vi "Main.vi"() -> ()   [LabVIEW 2017]
panel:
  out "spreadsheet string":string
  in  "Question 32":enum32{"1", "2", "3", "4", " IDK"}(radio)=enum." IDK"
  in  "Question 31":enum32{"1", "2", "3", "4", " IDK"}(radio)=enum." IDK"
  in  "Question 30":enum32{"1", "2", "3", "4", " IDK"}(radio)=enum." IDK"
  in  "Question 29":enum32{"1", "2", "3", "4", " IDK"}(radio)=enum." IDK"
  in  "Question 28":enum32{"1", "2", "3", "4", " IDK"}(radio)=enum." IDK"
  in  "Question 27":enum32{"1", "2", "3", "4", " IDK"}(radio)=enum." IDK"
  in  "Question 26":enum32{"1", "2", "3", "4", " IDK"}(radio)=enum." IDK"
  in  "Question 25":enum32{"1", "2", "3", "4", " IDK"}(radio)=enum." IDK"
  in  "Question 24":enum32{"1", "2", "3", "4", " IDK"}(radio)=enum." IDK"
  in  "Question 23":enum32{"1", "2", "3", "4", " IDK"}(radio)=enum." IDK"
  in  "Question 22":enum32{"1", "2", "3", "4", " IDK"}(radio)=enum." IDK"
  in  "Question 21":enum32{"1", "2", "3", "4", " IDK"}(radio)=enum." IDK"
  in  "Question 20":enum32{"1", "2", "3", "4", " IDK"}(radio)=enum." IDK"
  in  "Question 19":enum32{"1", "2", "3", "4", " IDK"}(radio)=enum." IDK"
  in  "Question 18":enum32{"1", "2", "3", "4", " IDK"}(radio)=enum." IDK"
  in  "Question 17":enum32{"1", "2", "3", "4", " IDK"}(radio)=enum." IDK"
  in  "Question 16":enum32{"1", "2", "3", "4", " IDK"}(radio)=enum." IDK"
  in  "Question 15":enum32{"1", "2", "3", "4", " IDK"}(radio)=enum." IDK"
  in  "Question 14":enum32{"1", "2", "3", "4", " IDK"}(radio)=enum." IDK"
  in  "Question 13":enum32{"1", "2", "3", "4", " IDK"}(radio)=enum." IDK"
  in  "Question 12":enum32{"1", "2", "3", "4", " IDK"}(radio)=enum." IDK"
  in  "Question 11":enum32{"1", "2", "3", "4", " IDK"}(radio)=enum." IDK"
  in  "Question 10":enum32{"1", "2", "3", "4", " IDK"}(radio)=enum." IDK"
  in  "Question 9":enum32{"1", "2", "3", "4", " IDK"}(radio)=enum." IDK"
  in  "Question 8":enum32{"1", "2", "3", "4", " IDK"}(radio)=enum." IDK"
  in  "Question 7":enum32{"1", "2", "3", "4", " IDK"}(radio)=enum." IDK"
  in  "Question 6":enum32{"1", "2", "3", "4", " IDK"}(radio)=enum." IDK"
  in  "Question 5":enum32{"1", "2", "3", "4", " IDK"}(radio)=enum." IDK"
  in  "Question 4":enum32{"1", "2", "3", "4", " IDK"}(radio)=enum." IDK"
  in  "Question 3":enum32{"1", "2", "3", "4", " IDK"}(radio)=enum." IDK"
  in  "Question 2":enum32{"1", "2", "3", "4", " IDK"}(radio)=enum." IDK"
  in  "VISA resource name":refnum<visa-resource-name>
  in  "Question 1":enum32{"1", "2", "3", "4", " IDK"}(radio)=enum." IDK"
  in  "OK":bool
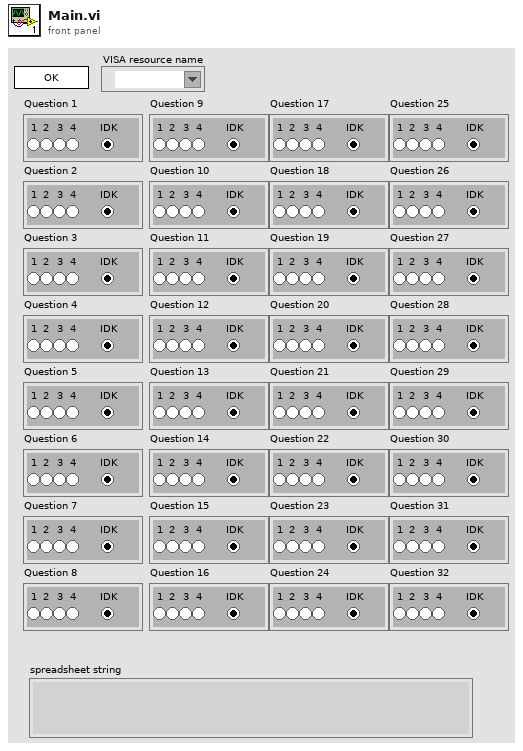
[diagram p1: front panel]
types:
  T1 = enum32{"invalid app kind", "Development System", "Run Time System", "Student Edition", "Embedded LabVIEW", "Evaluation", "Custom"}
  T2 = enum32{"Invalid", "Standard", "Closed", "Hidden", "Minimized", "Maximized"}
  T3 = cluster{"Core":cluster{"Current VI Reference":refnum<vi>, "Close Panel on Exit?":bool}, "Your Boolean data":bool, "Your string data":string, "resource name":refnum<visa-resource-name>}
  T4 = cluster{"Current VI Reference":refnum<vi>, "Close Panel on Exit?":bool}
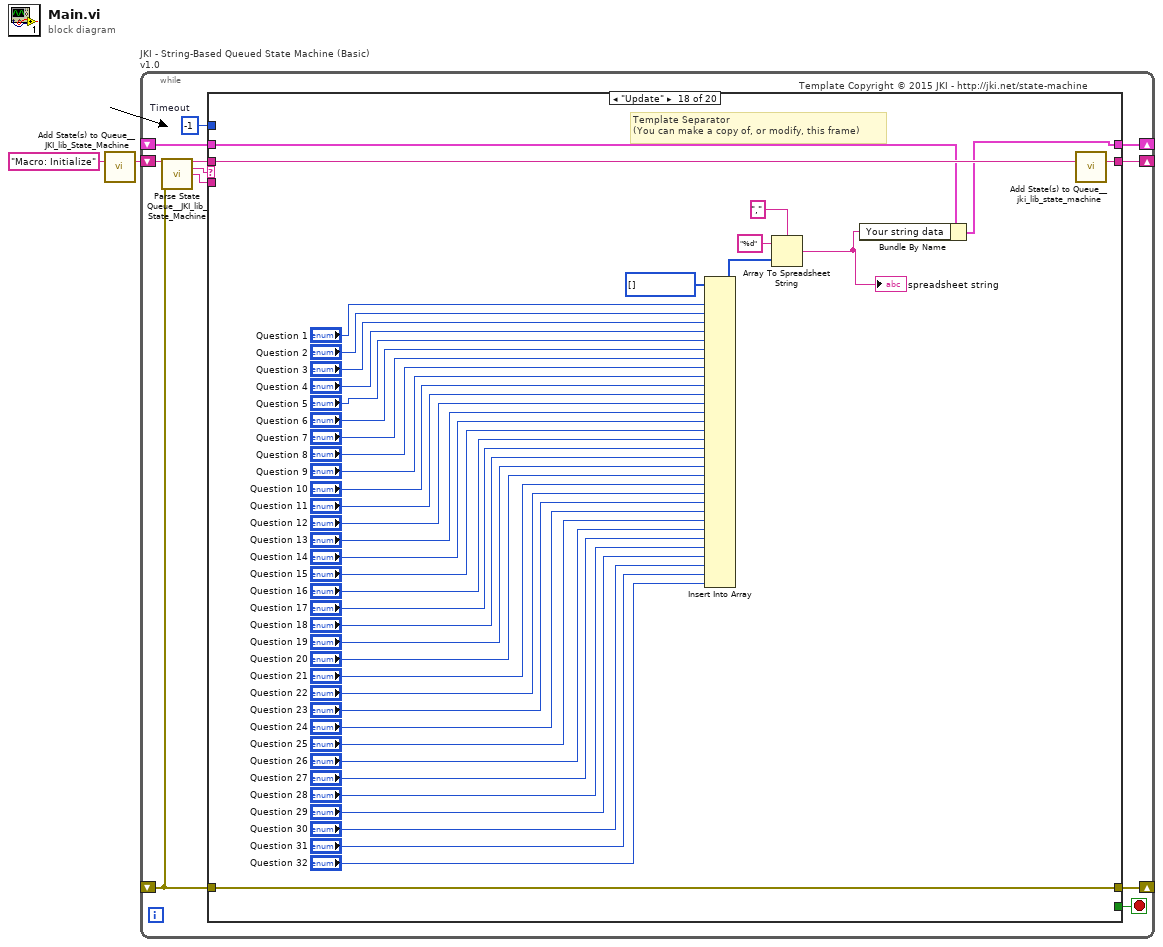
[diagram p0: block diagram]
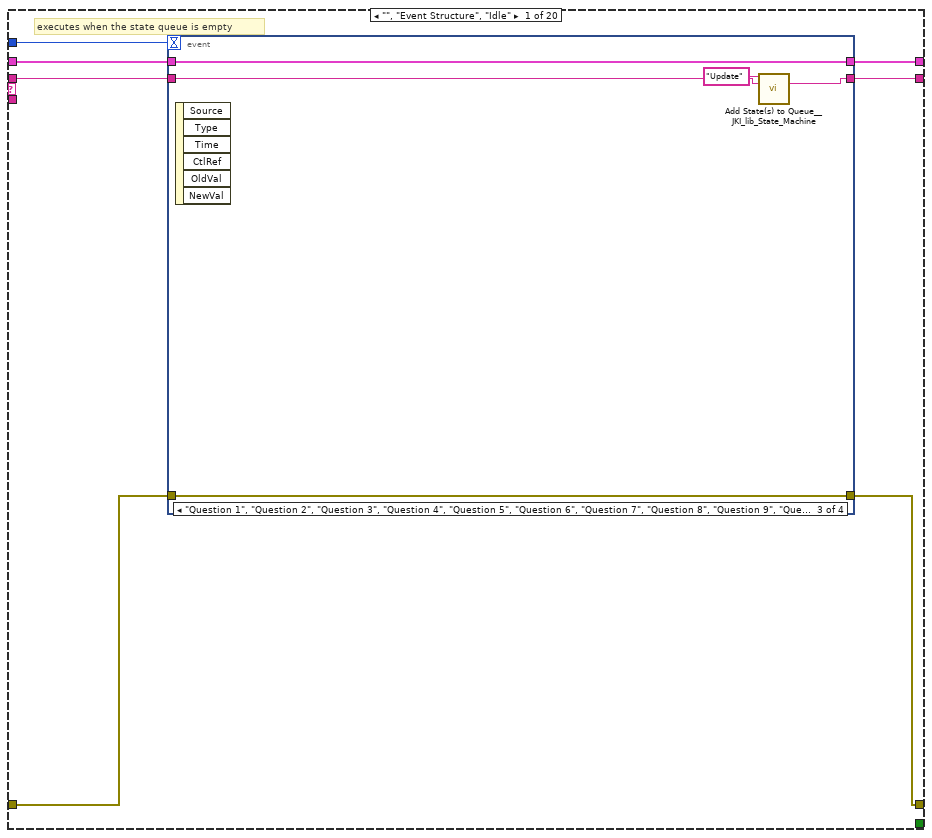
[diagram p2: hidden frame]
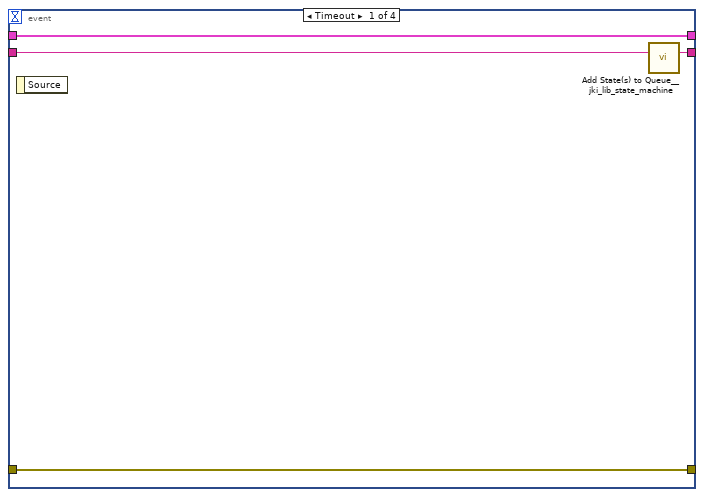
[diagram p3: hidden frame]
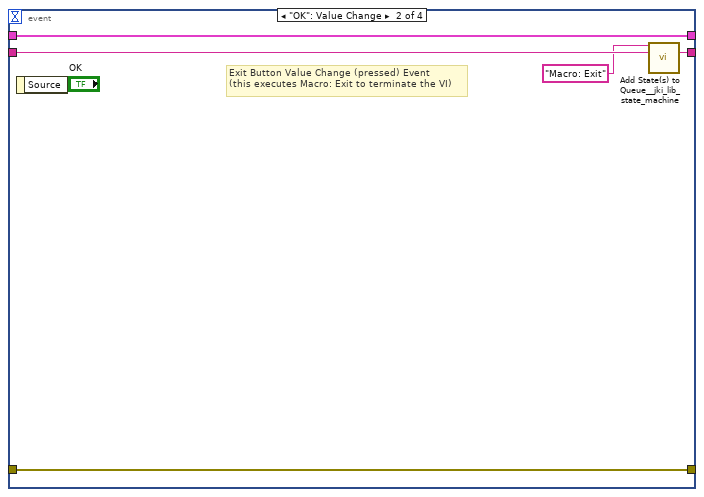
[diagram p4: hidden frame]
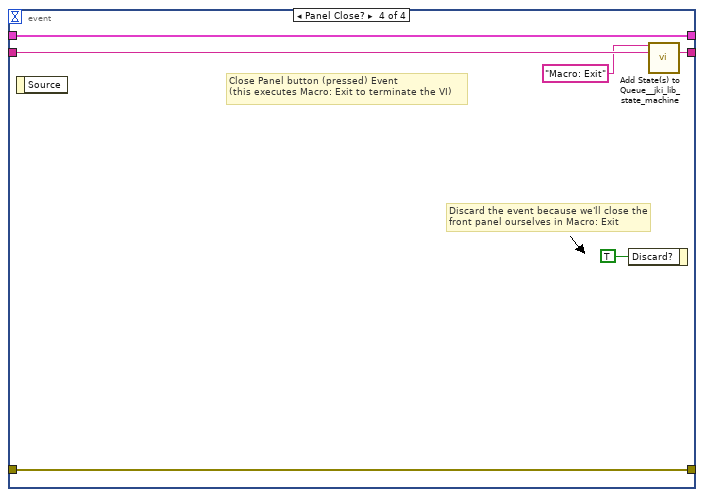
[diagram p5: hidden frame]
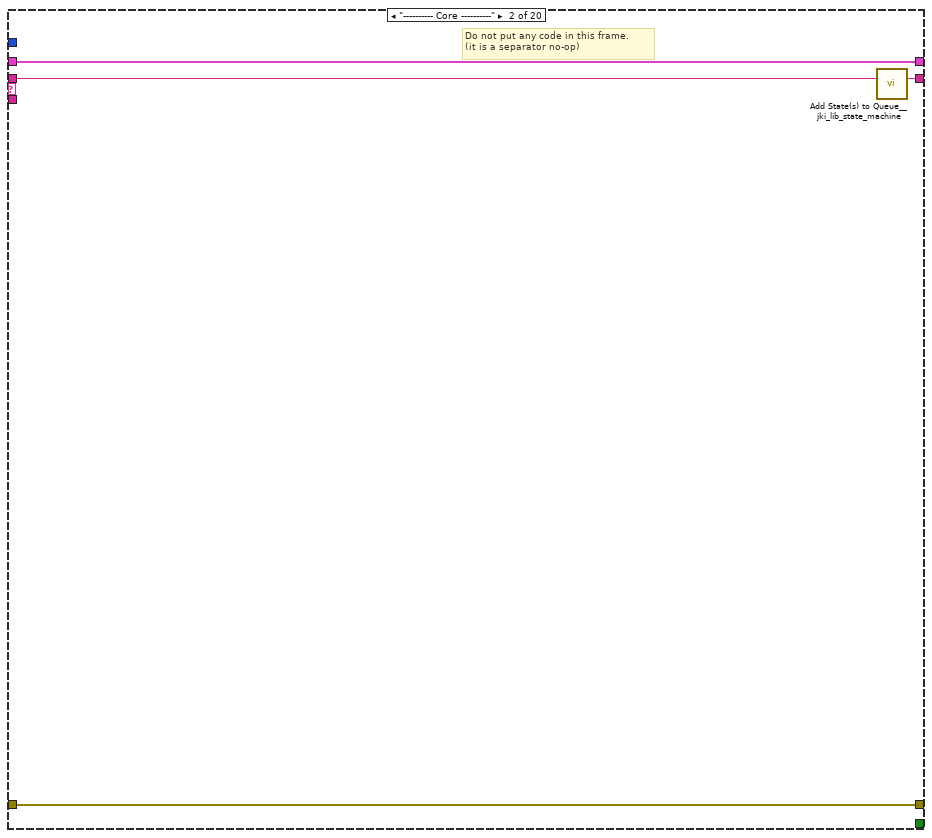
[diagram p6: hidden frame]
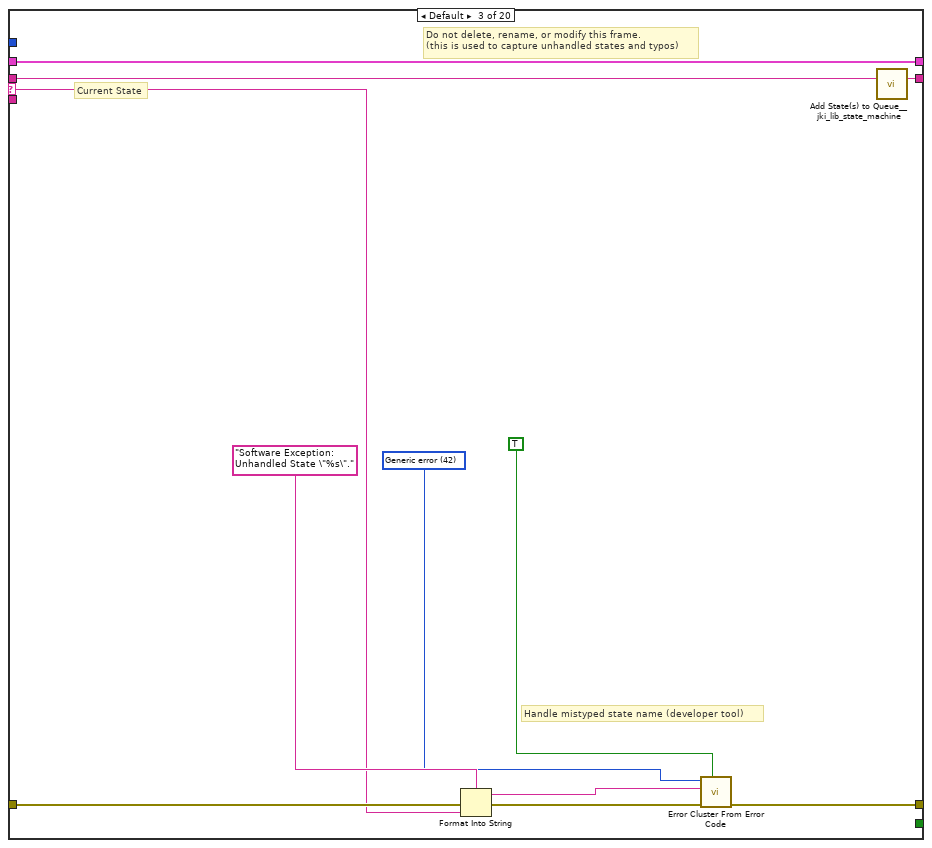
[diagram p7: hidden frame]
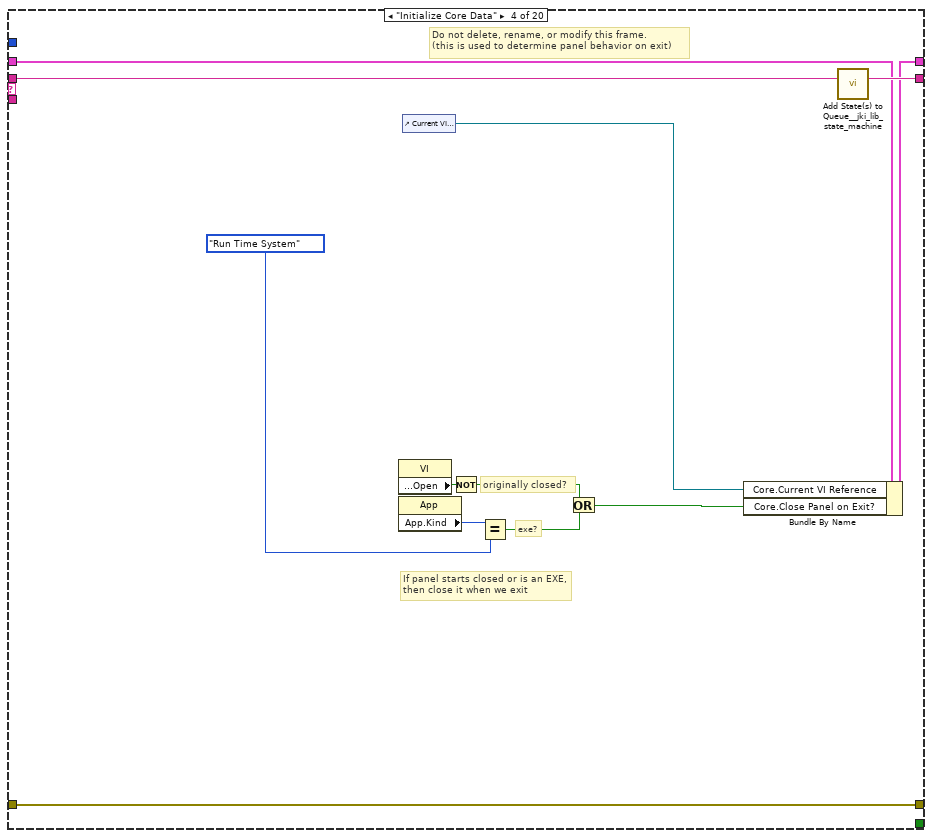
[diagram p8: hidden frame]
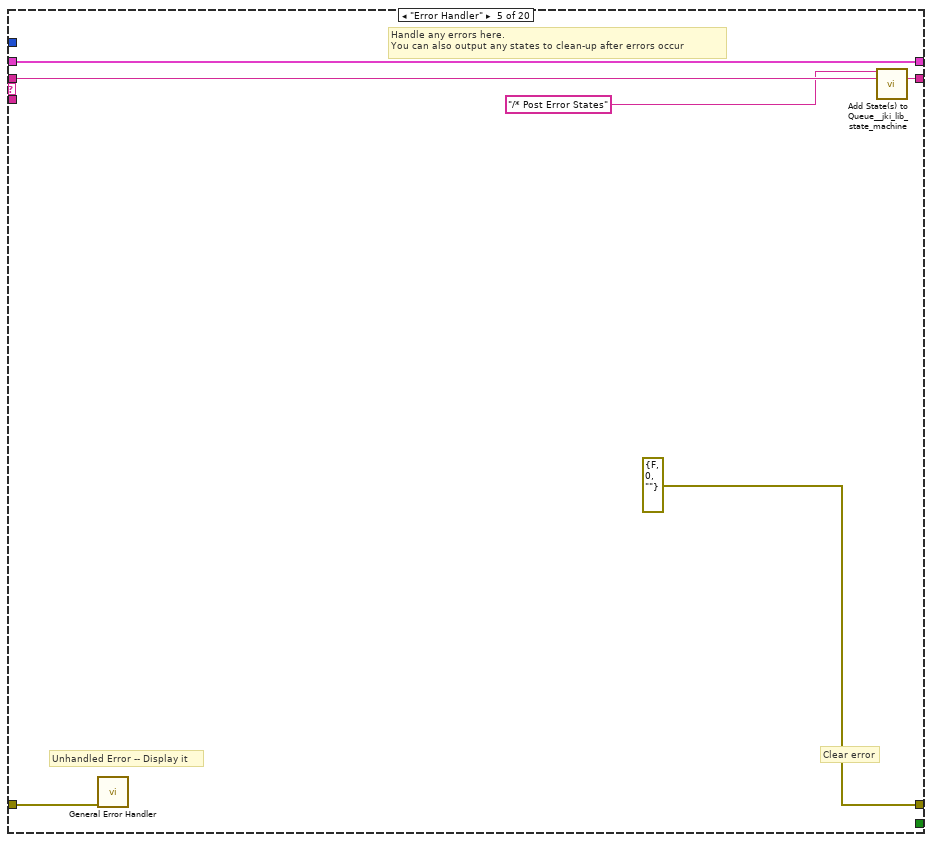
[diagram p9: hidden frame]
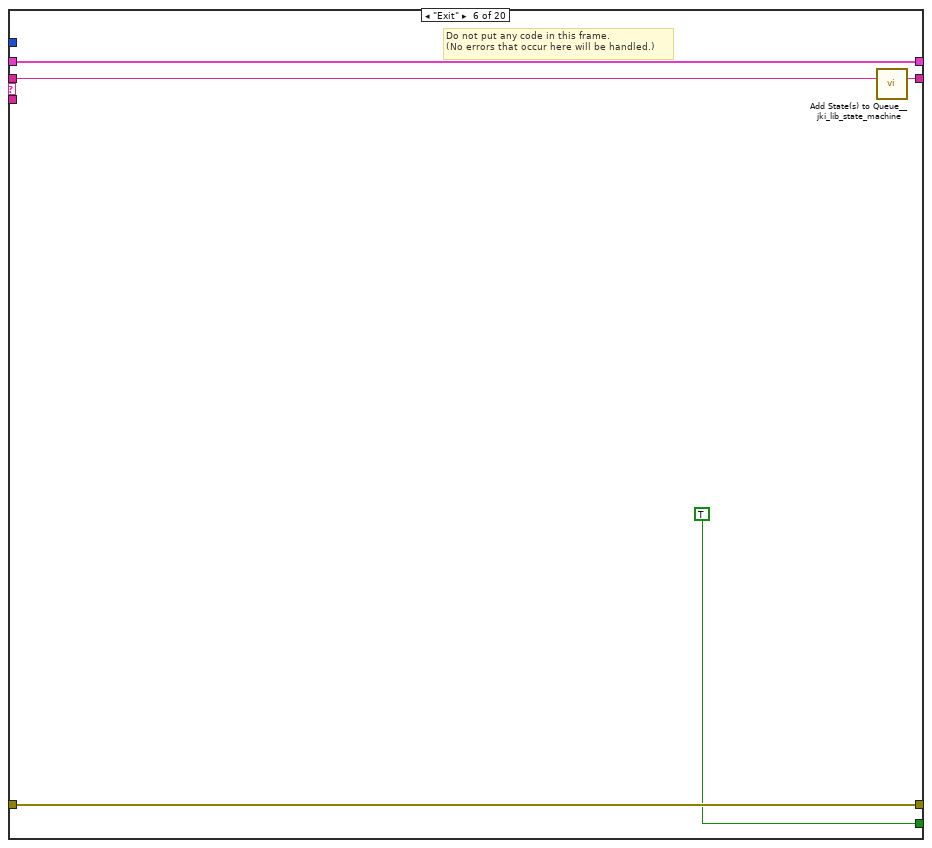
[diagram p10: hidden frame]
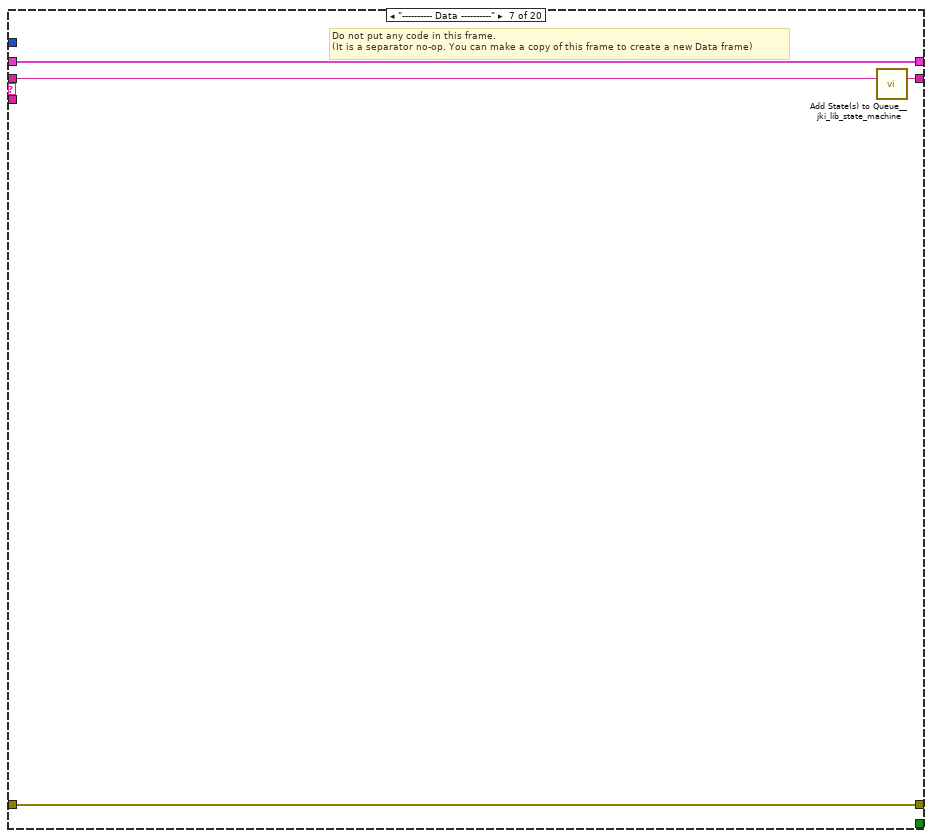
[diagram p11: hidden frame]
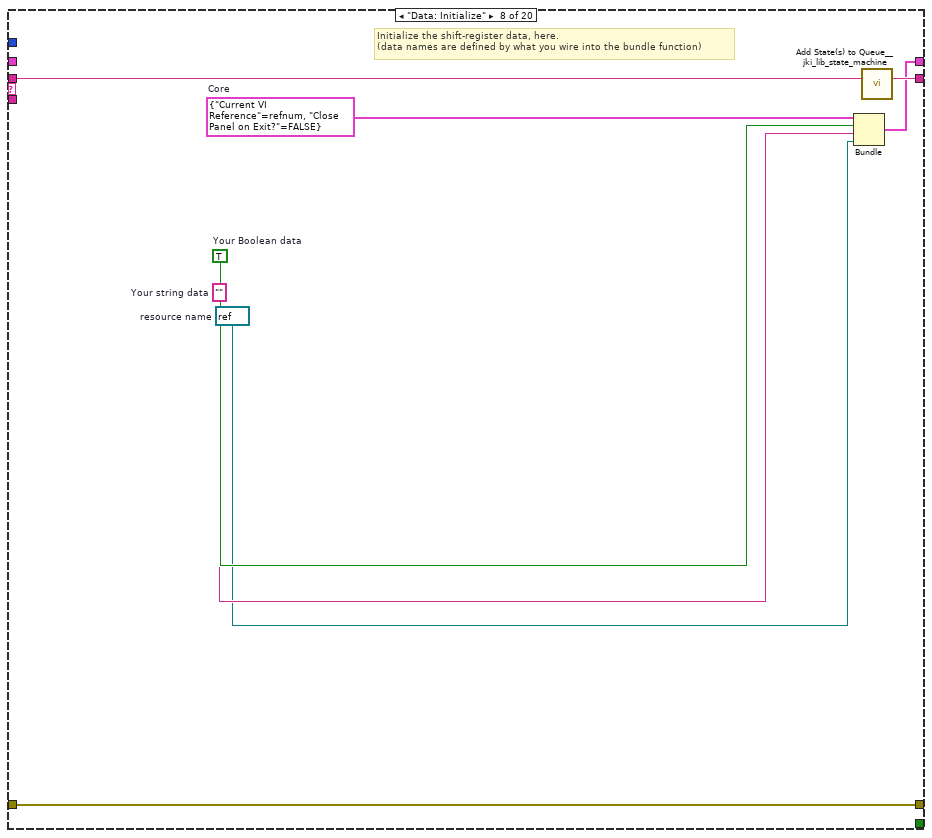
[diagram p12: hidden frame]
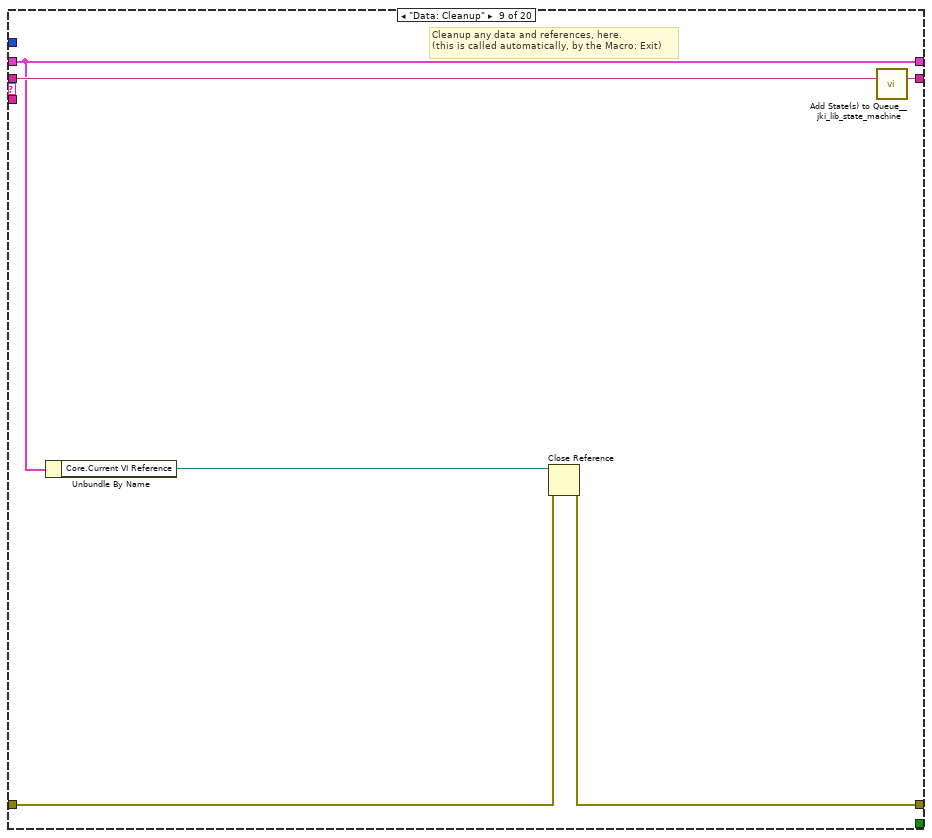
[diagram p13: hidden frame]
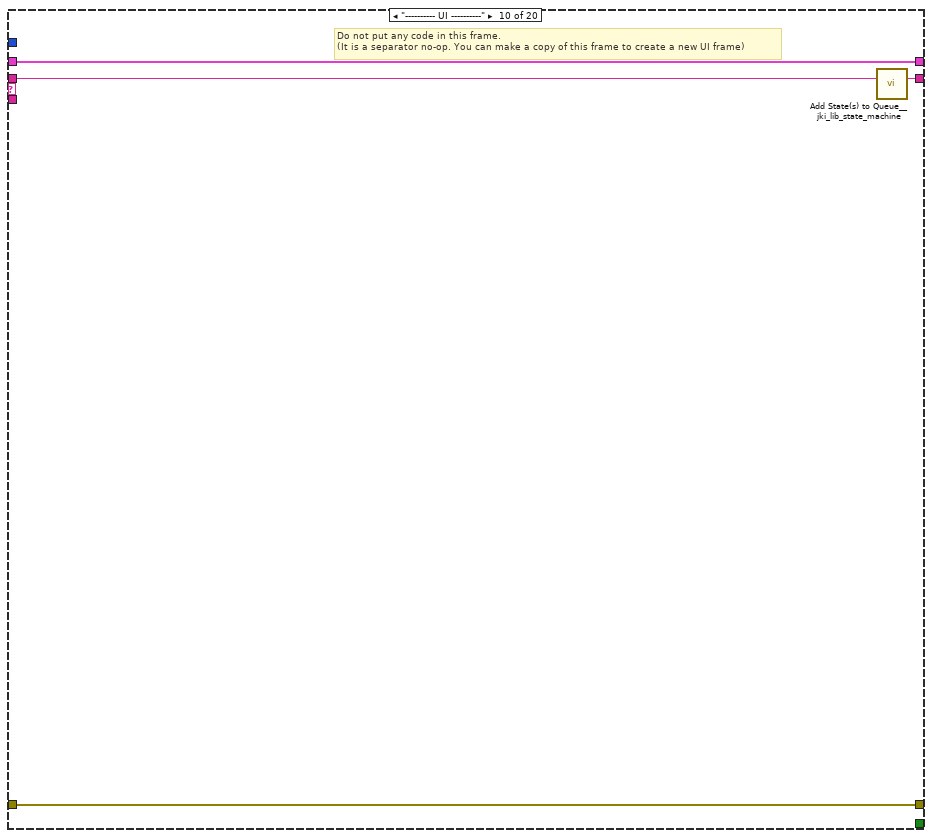
[diagram p14: hidden frame]
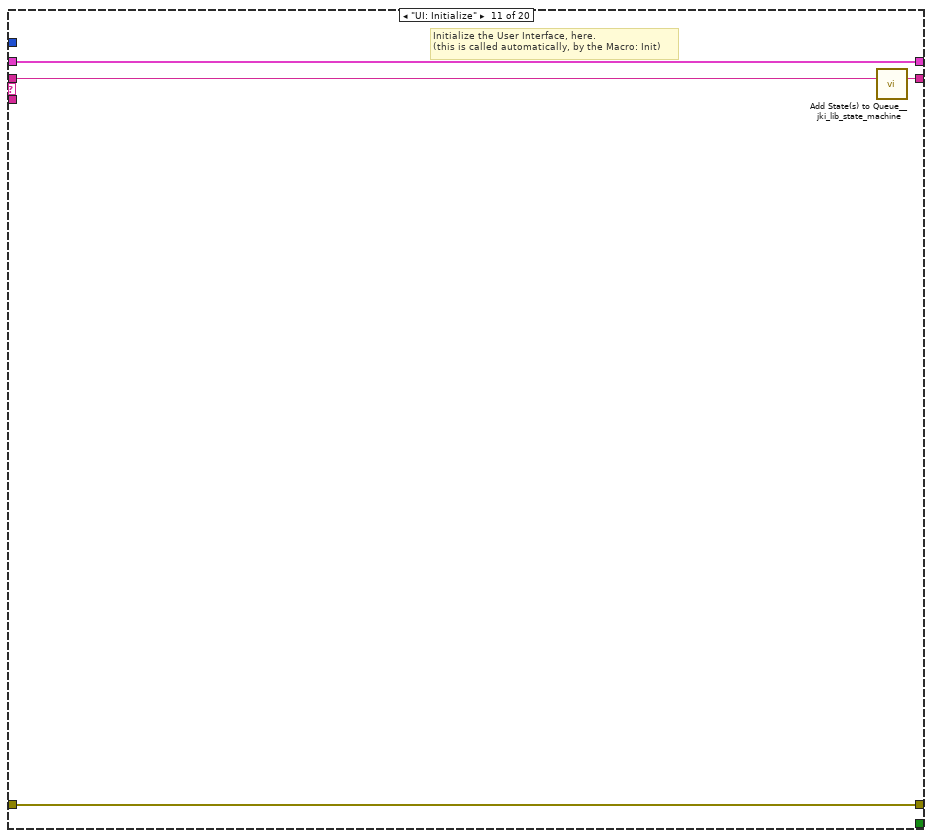
[diagram p15: hidden frame]
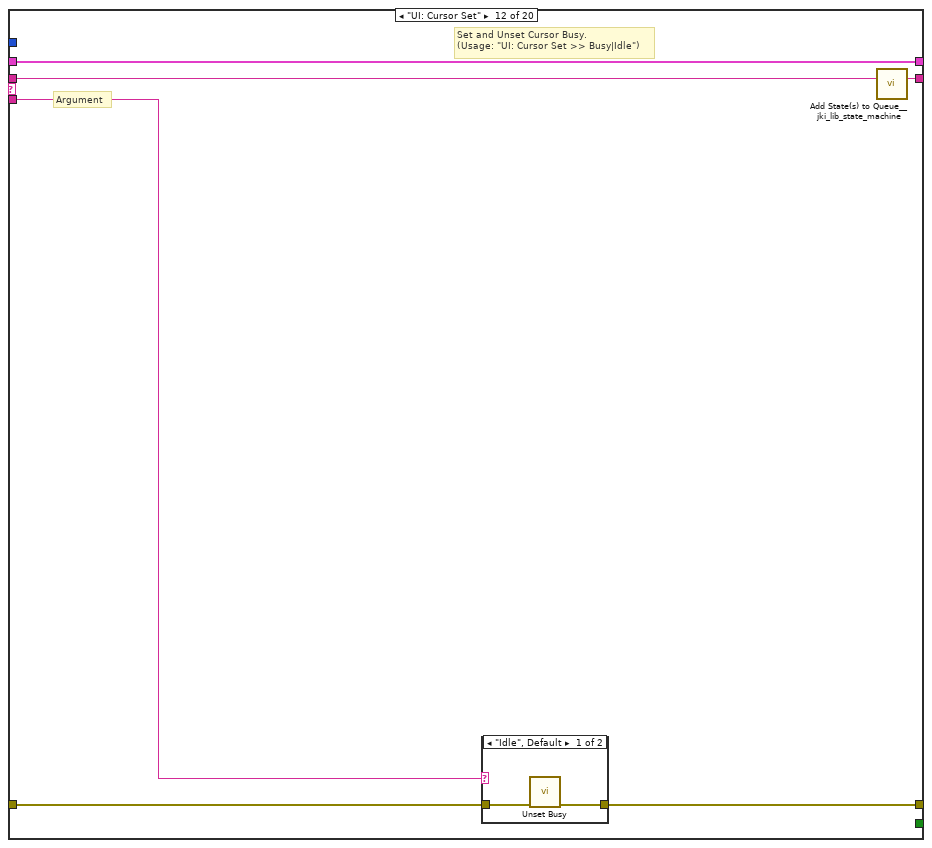
[diagram p16: hidden frame]
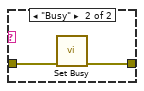
[diagram p17: hidden frame]
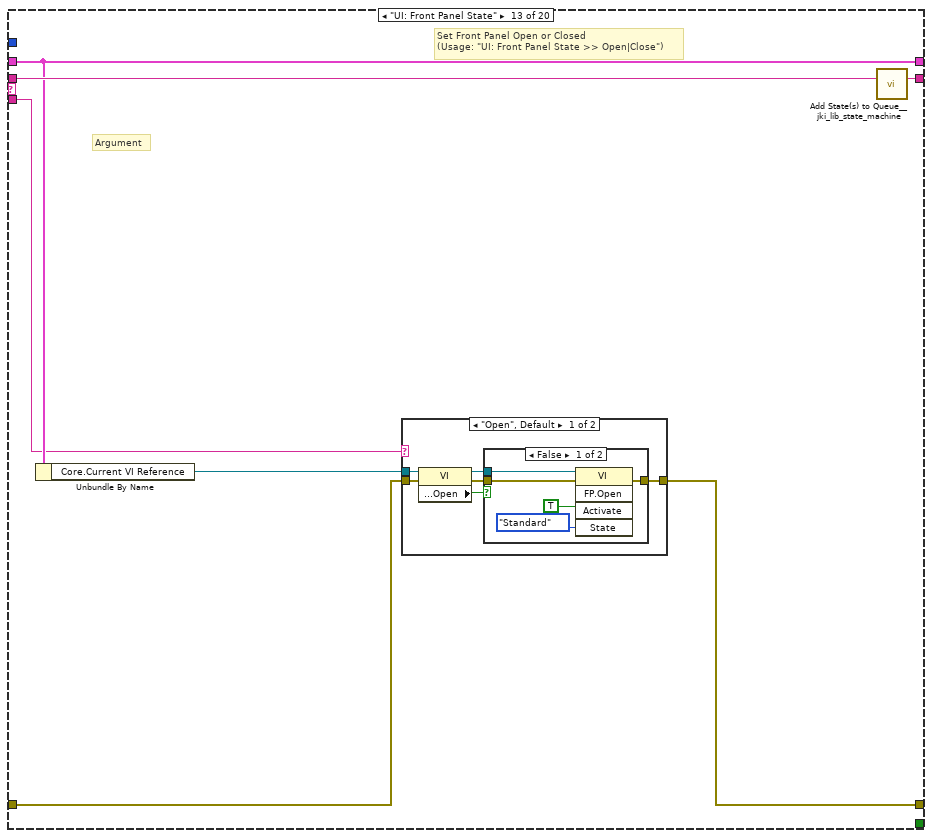
[diagram p18: hidden frame]
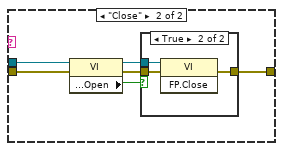
[diagram p20: hidden frame]
diagram:
  n1 = call <vilib>:"Add State(s) to Queue__JKI_lib_State_Machine.vi"("State(s) in (\"\")"="Macro: Initialize") -> ("States Out"=w2:string)  [unwired: 14 in]
  n2 = while "JKI - String-Based Queued State Machine (Basic) v1.0" {
    shift-right: [w6] -> _
    shift-left: _ -> [w5]
    shift-right: [w9] -> _
    shift-left: _ -> [w3]
    shift-right: [w8] -> _
    shift-left: w2 -> [w10]
    stop <- w7 stop-if-true
    w4 = -1  # Timeout
    # "Template Copyright © 2015 JKI - http://jki.net/state-machine"
    n3 = call <vilib>:"Parse State Queue__JKI_lib_State_Machine.vi"("State Queue"=w10, "Error In (no error)"=w3) -> ("Remaining States"=w12:string, "Current State"=w13:string, "Arguments"=w11:string)  [unwired: 11 in]
    n4 = case shown="\"Update\"" w13 {
      selector: w13 -> [_ _ w45 _ _ _ _ _ _ _ _ _ _ _ _ _ _ _ _ _]
      tunnel: w12 -> [w20 w44 w49 w67 w73 w78 w82 w90 w96 w100 w104 w110 w121 w147 w152 w162 w166 w208 w216 w223]
      tunnel: w11 -> [_ _ _ _ _ _ _ _ _ _ _ w105 w115 _ _ _ _ _ _ _]
      tunnel: w5 -> [w18 w41 w47 w58 w70 w76 w79 _ w91 w97 w102 w108 w117 w144 w149 w159 w163 w170 w212 w221]
      tunnel: [w17 w42 w51 w64 errorcluster {"status"=FALSE, "code"=0, "source"=""} ("error out") w75 w80 w87 w92 w98 w101 w106 w118 w145 w150 w160 w164 w206 w209 w218] -> w9
      tunnel: w3 -> [w16 w42 w50 w64 w69 w75 w80 w87 w93 w98 w101 w107 w119 w145 w150 w160 w164 w206 w210 w219]
      tunnel: [w19 w43 w48 w66 w72 w77 w81 w89 w95 w99 w103 w109 w120 w146 w151 w161 w165 w207 w215 w222] -> w8
      tunnel: [_ _ _ _ _ TRUE _ _ _ _ _ _ _ _ _ _ _ _ _ _] -> w7
      tunnel: [w15 w41 w47 w65 w70 w76 w79 w88 w91 w97 w102 w108 w117 w144 w149 w159 w163 w168 w213 w221] -> w6
      tunnel: w4 -> [w14 _ _ _ _ _ _ _ _ _ _ _ _ _ _ _ _ _ _ _]
      frame "", "Event Structure", "Idle" {
        # "executes when the state queue is empty"
        n5 = event shown="[2] \"Question 1\", \"Question 2\", \"Question 3\", \"Question 4\", \"Question 5\", \"Question 6\", \"Question 7\", \"Question 8\", \"Question 9\", \"Question 10\", \"Question 11\", \"Question 12\", \"Question 13\", \"Question 14\", \"Question 15\", \"Question 16\", \"Question 17\", \"Question 18\", \"Question 20\", \"Question 21\", \"Question 22\", \"Question 23\", \"Question 24\", \"Question 32\", \"Question 31\", \"Question 30\", \"Question 29\", \"Question 27\", \"Question 28\", \"Question 26\", \"Question 25\": Value Change" {
          selector: _ -> [_ _ _ _]
          dyn-events: _ -> [_ _ _ _]
          timeout: w14 -> [_ _ _ _]
          tunnel: w20 -> [w24 w29 w32 w40]
          tunnel: [w23 w28 w33 w39] -> w19
          tunnel: w18 -> [w21 w26 w34 w37]
          tunnel: [w22 w27 w30 w38] -> w17
          tunnel: w16 -> [w22 w27 w30 w38]
          tunnel: [w21 w26 w34 w37] -> w15
          event Timeout {
            n6 = event-data() -> ()  [unwired: 1 in, 1 out]
            n7 = call <vilib>:"Add State(s) to Queue__jki_lib_state_machine.vi"("State(s) in (\"\")"=w24) -> ("States Out"=w23:string)  [unwired: 14 in]
          }
          event "OK": Value Change {
            # "Exit Button Value Change (pressed) Event\n(this executes Macro: Exit to terminate the VI)"
            n8 = event-data() -> ()  [unwired: 1 in, 1 out]
            n9 = call <vilib>:"Add State(s) to Queue__jki_lib_state_machine.vi"("State(s) in Front (\"\")"="Macro: Exit", "State(s) in (\"\")"=w29) -> ("States Out"=w28:string)  [unwired: 13 in]
          }
          event "Question 1", "Question 2", "Question 3", "Question 4", "Question 5", "Question 6", "Question 7", "Question 8", "Question 9", "Question 10", "Question 11", "Question 12", "Question 13", "Question 14", "Question 15", "Question 16", "Question 17", "Question 18", "Question 20", "Question 21", "Question 22", "Question 23", "Question 24", "Question 32", "Question 31", "Question 30", "Question 29", "Question 27", "Question 28", "Question 26", "Question 25": Value Change {
            n10 = event-data() -> ()  [unwired: 1 in, 6 out]
            n11 = call <vilib>:"Add State(s) to Queue__JKI_lib_State_Machine.vi"("State(s) in Front (\"\")"="Update" ("State(s) in Front (\"\")"), "State(s) in (\"\")"=w32) -> ("States Out"=w33:string)  [unwired: 13 in]
          }
          event Panel Close? {
            # "Discard the event because we'll close the front panel ourselves in Macro: Exit"
            # "Close Panel button (pressed) Event\n(this executes Macro: Exit to terminate the VI)"
            n12 = event-data() -> ()  [unwired: 1 in, 1 out]
            n13 = event-data("Discard?"=TRUE) -> ()  [unwired: 1 in, 1 out]
            n14 = call <vilib>:"Add State(s) to Queue__jki_lib_state_machine.vi"("State(s) in Front (\"\")"="Macro: Exit", "State(s) in (\"\")"=w40) -> ("States Out"=w39:string)  [unwired: 13 in]
          }
        }
      }
      frame "---------- Core ----------" {
        # "Do not put any code in this frame.\n(it is a separator no-op)"
        n15 = call <vilib>:"Add State(s) to Queue__jki_lib_state_machine.vi"("State(s) in (\"\")"=w44) -> ("States Out"=w43:string)  [unwired: 14 in]
      }
      frame Default {
        w54 = 42 items=["No error", "Argument error", "Memory is full", "Out of zone", "End of file", "File already open", "Generic file I/O error", "File not found", "File permission error", "Disk is full", "Duplicate path", "Too many files open", "System feature not enabled", "Resource file not found", "Cannot add resource", "Resource not found", "Image not found", "Image memory error", "Pen does not exist", "Config type invalid", "Config token not found", "Config parse error", "Config memory error", "Bad external code format", "Bad external code offset", "External code not present", "Null window", "Destroy window error", "Null menu", "Print aborted", "Bad print record", "Print driver error", "Windows error during printing", "Memory error during printing", "Print dialog error", "Generic print error", "Invalid device refnum", "Device not found", "Device parameter error", "Device unit error", "Cannot open device", "Device call aborted", "Generic error", "Cancelled by user", "Object ID too low", "Object ID too high", "Object not in heap", "Unknown heap", "Unknown object (invalid DefProc)", "Unknown object (DefProc not in table)", "Message out of range", "Invalid (null) method", "Unknown message", "Manager call not supported", "Bad address", "Network operation in progress", "Network operation timed out", "Connection is busy", "Network attribute not supported", "Network error", "Address in use", "System out of memory", "Connection aborted", "Connection refused", "Not connected", "Already connected", "Connection closed", "Initialization error (interapplication manager)", "Bad occurrence", "Wait on unbound occurrence handler", "Occurrence queue overflow", "Datalog type conflict", "Unused", "Unrecognized type (interapplication manager)", "Memory corrupt", "Failed to make temporary DLL", "Old CIN version", "Drag socket not found", "Failed to load drop-object", "Failed to register OLE object", "Failed to release OLE object", "Format specifier type mismatch", "Unknown format specifier", "Too few format specifiers", "Too many format specifiers", "Scan failed", "Newer CIN version", "Error converting to variant", "Runtime menu error", "Password tampered", "Variant attribute not found", "Incompatible variant data type", "Event data is not available", "Event Store is not present", "Occurrence is not found", "Event Queue is not created", "Event info is not available", "Refnum passed is NULL", "Error retrieving Class GUID", "Error retrieving CoClass GUID", "Error retrieving TypeLib GUID.", "Bad built application magic bytes.", "Specific driver is different from the specific driver associated with the Logical Name.", "There is no session opened to the class driver.", "Max Error", "MAX - Error with config objects", "MAX - Error loading configuration", "MAX - Group not supported"]
        # "Current State"
        # "Do not delete, rename, or modify this frame.\n(this is used to capture unhandled states and typos)"
        # "Handle mistyped state name (developer tool)"
        n16 = Format Into String(format string="Software Exception: Unhandled State \"%s\"." ("message"), error in=w50, w45) -> (resulting string=w53:string, error out=w52:errorcluster)  [unwired: 1 in]
        n17 = call <vilib>:"Error Cluster From Error Code.vi"("show call chain? (False)"=TRUE, "error in (no error)"=w52, "error message (\"\")"=w53, "error code (0)"=w54) -> ("error out"=w51:errorcluster)  [unwired: 5 in]
        n18 = call <vilib>:"Add State(s) to Queue__jki_lib_state_machine.vi"("State(s) in (\"\")"=w49) -> ("States Out"=w48:string)  [unwired: 14 in]
      }
      frame "Initialize Core Data" {
        # "Do not delete, rename, or modify this frame.\n(this is used to determine panel behavior on exit)"
        # "originally closed?"
        # "exe?"
        # "If panel starts closed or is an EXE, then close it when we exit"
        n19 = property class="VI"() -> ("Front Panel.Open"=w63:bool)  [unwired: 2 in, 2 out]
        n20 = property class="App"() -> ("App.Kind"=w62:T1)  [unwired: 2 in, 2 out]
        n21 = control-ref of="Current VI Reference"() -> (w56:refnum<vi>)
        n22 = Not(x=w63) -> (.not. x?=w60:bool)
        n23 = Equal?(x=w62, y=T1."Run Time System" ("Application:Kind")) -> (x = y?=w59:bool)
        n24 = Or(x=w60, y=w59) -> (x .or. y?=w57:bool)
        n25 = Bundle By Name(cluster=w58, "Core.Current VI Reference"=w56, "Core.Close Panel on Exit?"=w57) -> (w65:T3)
        n26 = call <vilib>:"Add State(s) to Queue__jki_lib_state_machine.vi"("State(s) in (\"\")"=w67) -> ("States Out"=w66:string)  [unwired: 14 in]
      }
      frame "Error Handler" {
        # "Unhandled Error -- Display it"
        # "Handle any errors here.\nYou can also output any states to clean-up after errors occur"
        # "Clear error"
        n27 = call <vilib>:"General Error Handler.vi"("error in (no error)"=w69) -> ()  [unwired: 10 in, 5 out]
        n28 = call <vilib>:"Add State(s) to Queue__jki_lib_state_machine.vi"("State(s) in Front (\"\")"="/* Post Error States", "State(s) in (\"\")"=w73) -> ("States Out"=w72:string)  [unwired: 13 in]
      }
      frame "Exit" {
        # "Do not put any code in this frame.\n(No errors that occur here will be handled.)"
        n29 = call <vilib>:"Add State(s) to Queue__jki_lib_state_machine.vi"("State(s) in (\"\")"=w78) -> ("States Out"=w77:string)  [unwired: 14 in]
      }
      frame "---------- Data ----------" {
        # "Do not put any code in this frame.\n(It is a separator no-op. You can make a copy of this frame to create a new Data frame)"
        n30 = call <vilib>:"Add State(s) to Queue__jki_lib_state_machine.vi"("State(s) in (\"\")"=w82) -> ("States Out"=w81:string)  [unwired: 14 in]
      }
      frame "Data: Initialize" {
        w83 = refnum<visa-resource-name> refnum  # resource name
        w84 = T4 {"Current VI Reference"=refnum, "Close Panel on Exit?"=FALSE}  # Core
        w86 = TRUE  # Your Boolean data
        w85 = ""  # Your string data
        # "Initialize the shift-register data, here.\n(data names are defined by what you wire into the bundle function)"
        n31 = Bundle("Core"=w84, "Your Boolean data"=w86, "Your string data"=w85, "resource name"=w83) -> (w88:T3)  [unwired: 1 in]
        n32 = call <vilib>:"Add State(s) to Queue__jki_lib_state_machine.vi"("State(s) in (\"\")"=w90) -> ("States Out"=w89:string)  [unwired: 14 in]
      }
      frame "Data: Cleanup" {
        # "Cleanup any data and references, here.\n(this is called automatically, by the Macro: Exit)"
        n33 = Unbundle By Name(w91) -> ("Core.Current VI Reference"=w94:refnum<vi>)
        n34 = Close Reference(reference=w94, error in (no error)=w93) -> (error out=w92:errorcluster)
        n35 = call <vilib>:"Add State(s) to Queue__jki_lib_state_machine.vi"("State(s) in (\"\")"=w96) -> ("States Out"=w95:string)  [unwired: 14 in]
      }
      frame "---------- UI ----------" {
        # "Do not put any code in this frame.\n(It is a separator no-op. You can make a copy of this frame to create a new UI frame)"
        n36 = call <vilib>:"Add State(s) to Queue__jki_lib_state_machine.vi"("State(s) in (\"\")"=w100) -> ("States Out"=w99:string)  [unwired: 14 in]
      }
      frame "UI: Initialize" {
        # "Initialize the User Interface, here.\n(this is called automatically, by the Macro: Init)"
        n37 = call <vilib>:"Add State(s) to Queue__jki_lib_state_machine.vi"("State(s) in (\"\")"=w104) -> ("States Out"=w103:string)  [unwired: 14 in]
      }
      frame "UI: Cursor Set" {
        # "Argument"
        # "Set and Unset Cursor Busy.\n(Usage: \"UI: Cursor Set >> Busy|Idle\")"
        n38 = case shown="\"Idle\", Default" w105 {
          tunnel: w107 -> [w112 w114]
          tunnel: [w111 w113] -> w106
          frame "Idle", Default {
            n39 = call <vilib>:"Unset Busy.vi"("error in (no error)"=w112) -> ("error out"=w111:errorcluster)  [unwired: 10 in]
          }
          frame "Busy" {
            n40 = call <vilib>:"Set Busy.vi"("error in (no error)"=w114) -> ("error out"=w113:errorcluster)  [unwired: 9 in, 1 out]
          }
        }
        n41 = call <vilib>:"Add State(s) to Queue__jki_lib_state_machine.vi"("State(s) in (\"\")"=w110) -> ("States Out"=w109:string)  [unwired: 14 in]
      }
      frame "UI: Front Panel State" {
        # "Argument"
        # "Set Front Panel Open or Closed\n(Usage: \"UI: Front Panel State >> Open|Close\")"
        n42 = Unbundle By Name(w117) -> ("Core.Current VI Reference"=w116:refnum<vi>)
        n43 = case shown="\"Open\", Default" w115 {
          tunnel: w119 -> [w125 w138]
          tunnel: [w127 w139] -> w118
          tunnel: w116 -> [w126 w136]
          frame "Open", Default {
            n44 = property class="VI"(reference=w126, error in=w125) -> (reference out=w123:refnum<vi>, error out=w124:errorcluster, "Front Panel.Open"=w122:bool)
            n45 = case shown="False" w122 {
              tunnel: [w130 w133] -> w127
              tunnel: w124 -> [w129 w133]
              tunnel: w123 -> [w128 _]
              frame False {
                n46 = invoke class="VI" method="FP.Open"(reference=w128, error in=w129, "Activate"=TRUE, "State"=T2."Standard") -> (error out=w130:errorcluster)  [unwired: 1 in, 4 out]
              }
              frame True {
              }
            }
          }
          frame "Close" {
            n47 = property class="VI"(reference=w136, error in=w138) -> (reference out=w135:refnum<vi>, error out=w137:errorcluster, "Front Panel.Open"=w134:bool)
            n48 = case shown="True" w134 {
              tunnel: [w140 w143] -> w139
              tunnel: w137 -> [w140 w142]
              tunnel: w135 -> [_ w141]
              frame False {
              }
              frame True {
                n49 = invoke class="VI" method="FP.Close"(reference=w141, error in=w142) -> (error out=w143:errorcluster)  [unwired: 1 in, 2 out]
              }
            }
          }
        }
        n50 = call <vilib>:"Add State(s) to Queue__jki_lib_state_machine.vi"("State(s) in (\"\")"=w121) -> ("States Out"=w120:string)  [unwired: 14 in]
      }
      frame "---------- Macro ----------" {
        # "Do not put any code in this frame.\n(It is a separator no-op. You can make a copy of this frame to create a new Macro frame)"
        n51 = call <vilib>:"Add State(s) to Queue__jki_lib_state_machine.vi"("State(s) in (\"\")"=w147) -> ("States Out"=w146:string)  [unwired: 14 in]
      }
      frame "Macro: Initialize" {
        w148 = "Data: Initialize\nInitialize Core Data\nUI: Initialize\nUI: Front Panel State >> Open"  # Data: Initialize Initialize Core Data UI: Initialize UI: Front Panel State >> Open
        # "Initialization Macro\n(This is called once, when the VI starts)"
        n52 = call <vilib>:"Add State(s) to Queue__jki_lib_state_machine.vi"("State(s) in Front (\"\")"=w148, "State(s) in (\"\")"=w152) -> ("States Out"=w151:string)  [unwired: 13 in]
      }
      frame "Macro: Exit" {
        # "Exit Macro\n(This is called once, when the VI exits)"
        n53 = Unbundle By Name(w159) -> ("Core.Close Panel on Exit?"=w158:bool)
        n54 = Select(t="UI: Front Panel State >> Close", s=w158, f="") -> (s? t:f=w155:string)
        n55 = call <vilib>:"Add State(s) to Queue__jki_lib_state_machine.vi"("State(s) in (\"\")"=w155, "State(s) at Back (\"\")"="Data: Cleanup\nExit") -> ("States Out"=w153:string)  [unwired: 13 in]
        n56 = call <vilib>:"Add State(s) to Queue__jki_lib_state_machine.vi"("State(s) in Front (\"\")"=w153, "State(s) in (\"\")"=w162) -> ("States Out"=w161:string)  [unwired: 13 in]
      }
      frame "---------- New Category ----------" {
        # "Template Separator\n(You can make a copy of, or modify, this frame)"
        n57 = call <vilib>:"Add State(s) to Queue__jki_lib_state_machine.vi"("State(s) in (\"\")"=w166) -> ("States Out"=w165:string)  [unwired: 14 in]
      }
      frame "Update" {
        w167 = enum32{"1", "2", "3", "4", " IDK"}[] [] items=["1", "2", "3", "4", " IDK"] ("array")
        # "Template Separator\n(You can make a copy of, or modify, this frame)"
        n58 = Insert Into Array(array=w167, new element #1="Question 1", new element #2="Question 2", new element #3="Question 3", new element #4="Question 4", new element #5="Question 5", new element #6="Question 6", new element #7="Question 7", new element #8="Question 8", new element #9="Question 9", new element #10="Question 10", new element #11="Question 11", new element #12="Question 12", new element #13="Question 13", new element #14="Question 14", new element #15="Question 15", new element #16="Question 16", new element #17="Question 17", new element #18="Question 18", new element #19="Question 19", new element #20="Question 20", new element #21="Question 21", new element #22="Question 22", new element #23="Question 23", new element #24="Question 24", new element #25="Question 25", new element #26="Question 26", new element #27="Question 27", new element #28="Question 28", new element #29="Question 29", new element #30="Question 30", new element #31="Question 31", new element #32="Question 32") -> (w205:enum32{"1", "2", "3", "4", " IDK"}[])  [unwired: 1 in]
        n59 = Array To Spreadsheet String(delimiter (Tab)=",", array=w205, 3:"%d" ("format string")) -> (spreadsheet string=w169:string)
        "spreadsheet string" <- w169
        n60 = Bundle By Name(cluster=w170, "Your string data"=w169) -> (w168:T3)
        n61 = call <vilib>:"Add State(s) to Queue__jki_lib_state_machine.vi"("State(s) in (\"\")"=w208) -> ("States Out"=w207:string)  [unwired: 14 in]
      }
      frame "SetComm: 1" {
        # "Your code here.\n(You can make a copy of, or modify, this frame)"
        n62 = VISA Open(error in (no error)=w210, VISA resource name="VISA resource name") -> (VISA resource name=w211:refnum<visa-resource-name>, error out=w209:errorcluster)  [unwired: 3 in]
        n63 = Bundle By Name(cluster=w212, "resource name"=w211) -> (w213:T3)
        n64 = call <vilib>:"Add State(s) to Queue__jki_lib_state_machine.vi"("State(s) in (\"\")"=w216) -> ("States Out"=w215:string)  [unwired: 14 in]
      }
      frame "Write : 2" {
        # "Your code here.\n(You can make a copy of, or modify, this frame)"
        n65 = Unbundle By Name(w221) -> ("resource name"=w220:refnum<visa-resource-name>, "Your string data"=w217:string)
        n66 = VISA Write(VISA resource name=w220, write buffer=w217, error in (no error)=w219) -> (error out=w218:errorcluster)  [unwired: 2 out]
        n67 = call <vilib>:"Add State(s) to Queue__jki_lib_state_machine.vi"("State(s) in (\"\")"=w223) -> ("States Out"=w222:string)  [unwired: 14 in]
      }
    }
  }
